vi "SndPB - Start.vi"(0 "reference in":refnum<class "GSwFormDSP.lvclass">, 5 "error in (no error)":errorcluster, 7 "Cursor Init Location (s)":dbl, 9 "Normalization Option":T1(ring)=enum."To itself", 11 "Signal Index":i32, 13 "SC Volume":dbl(slide)=100.0 caption="Volume" scale=0.0..100.0) -> (14 "reference out":refnum<class "GSwFormDSP.lvclass">, 19 "error out":errorcluster)   [LabVIEW 2022 SP3, in "GSwFormDSP.lvclass"]
uses:
  GSwFormDSP.lvclass
  <vilib>/sound2/lvsound2.llb/Sampling Mode.ctl
  <vilib>/sound2/lvsound2.llb/Sound Data Format.ctl
  <vilib>/sound2/lvsound2.llb/Sound Output Set Volume (Single).vi
  <vilib>/sound2/lvsound2.llb/Sound Output Write (DBL Single).vi
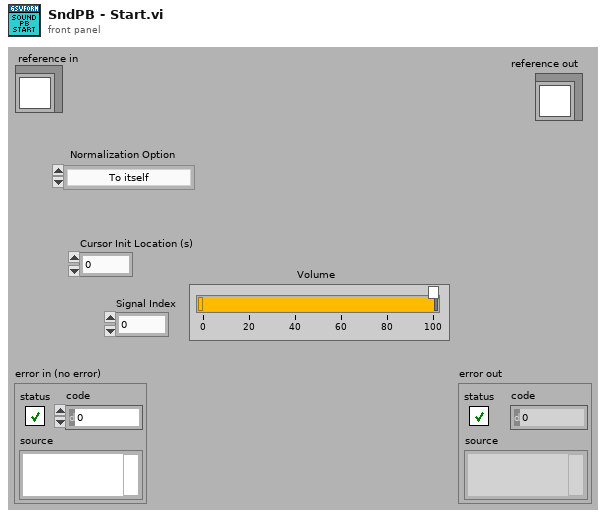
[diagram p1: front panel]
types:
  T1 = enum16{"None", "To itself", "To the max levels of ALL the signals"}
  T2 = typedef "Sound Data Format.ctl" = cluster{"sample rate (S/s)":dbl, "number of channels":i32, "bits per sample":i32}
  T3 = enum16{"Fade IN and OUT", "Fade IN ONLY", "Fade OUT ONLY", "None"}
  T4 = typedef "Sampling Mode.ctl" = i32
  T5 = typedef "Sound Output Task ID.ctl" = u32
  T6 = typedef "GSwFormDSP.lvclass/Sound Playback.ctl" = cluster{"Timer start (ms)":u32, "task ID":T5, "Cursor Init Location (s)":dbl, "SC Volume":dbl}
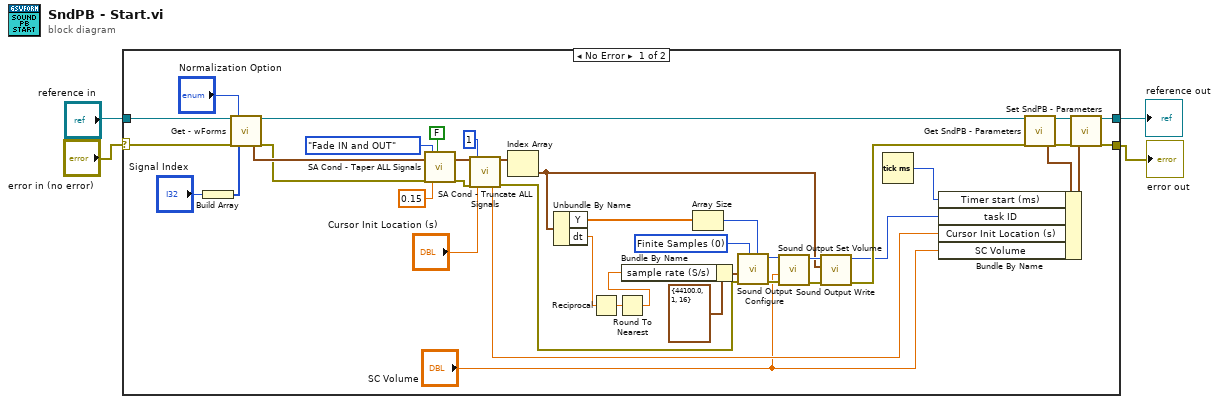
[diagram p0: block diagram]
diagram:
  n1 = case shown="No Error" "error in (no error)" {
    selector: "error in (no error)" -> [w9 w47]
    tunnel: [w18 w47] -> w3
    tunnel: [w19 w46] -> w1
    tunnel: "reference in" -> [w8 w46]
    frame No Error {
      w34 = T4 0 items=["Finite Samples", "Continuous Samples"] ("sample mode")
      n2 = Build Array("Signal Index") -> (w25:i32[])
      n3 = call-dynamic "Get - wForms.vi"("reference in"=w8, "error in (no error)"=w9, "Normalization Option"="Normalization Option", "Indexes (Empty = ALL)"=w25) -> ("wForms"=w23:waveform(dbl)[], "reference out"=w22:refnum<class "GSwFormDSP.lvclass">, "error out"=w12:errorcluster)  [unwired: 12 in, 1 out]
      n4 = call "SA Cond - Taper ALL Signals.vi"("wForm IN"=w23, "error in (no error)"=w12, "Fade Options"=T3."Fade IN and OUT", "Time for Fade IN/OUT (sec)"=0.15, "Anotate Signal Name"=FALSE) -> ("wForm OUT"=w45:waveform(dbl)[], "error out"=w43:errorcluster)  [unwired: 13 in]
      n5 = call "SA Cond - Truncate ALL Signals.vi"("wForm IN"=w45, "error in (no error)"=w43, "Nb Signals"=1, "Start (sec)"="Cursor Init Location (s)") -> ("actual start samples/time"=w6:dbl, "wForm OUT"=w41:waveform(dbl)[], "error out"=w26:errorcluster)  [unwired: 12 in, 1 out]
      n6 = Index Array(array=w41) -> (element=w27:waveform(dbl))  [unwired: 1 in]
      n7 = Unbundle By Name(w27) -> ("Y"=w31:dbl[], "dt"=w32:dbl)
      n8 = Reciprocal(x=w32) -> (1/x=w38:dbl)
      n9 = Round To Nearest(number=w38) -> (nearest integer value=w39:dbl)
      n10 = Bundle By Name(cluster=T2 {"sample rate (S/s)"=44100.0, "number of channels"=1, "bits per sample"=16} ("sound format"), "sample rate (S/s)"=w39) -> (w37:T2)
      n11 = Array Size(array=w31) -> (size(s)=w30:i32)
      n12 = call <vilib>:"Sound Output Configure.vi"("number of samples/ch"=w30, "sample mode"=w34, "error in (no error)"=w26, "sound format"=w37) -> ("error out"=w35:errorcluster, "task ID"=w36:T5)  [unwired: 6 in]
      n13 = call-poly <vilib>:"Sound Output Set Volume.vi"("error in (no error)"=w35, "volume"="SC Volume", "task ID"=w36) -> ("error out"=w28:errorcluster, "task ID out"=w29:T5)  [unwired: 7 in]
      n14 = call-poly <vilib>:"Sound Output Write.vi"("error in (no error)"=w28, "data"=w27, "task ID"=w29) -> ("error out"=w21:errorcluster, "task ID out"=w13:T5)  [unwired: 7 in]
      n15 = Tick Count (ms)() -> (millisecond timer value=w14:u32)
      n16 = call "Get SndPB - Parameters.vi"("reference in"=w22, "error in (no error)"=w21) -> ("Sound Playback"=w16:T6, "reference out"=w20:refnum<class "GSwFormDSP.lvclass">, "error out"=w17:errorcluster)  [unwired: 15 in]
      n17 = Bundle By Name(cluster=w16, "Timer start (ms)"=w14, "task ID"=w13, "Cursor Init Location (s)"=w6, "SC Volume"="SC Volume") -> (w15:T6)
      n18 = call "Set SndPB - Parameters.vi"("reference in"=w20, "error in (no error)"=w17, "Sound Playback"=w15) -> ("reference out"=w19:refnum<class "GSwFormDSP.lvclass">, "error out"=w18:errorcluster)  [unwired: 15 in]
    }
    frame Error {
    }
  }
  "error out" <- w3
  "reference out" <- w1
